vi "TestAsyncGrip.vi"() -> ()   [LabVIEW 2017]
uses:
  Projekt-RubikLibrary/ServoEnumControl.ctl
  Projekt-RubikLibrary/RubikLibraryRT.lvlib
  Projekt-RubikLibrary/RubikLibrary.lvlib
panel:
  in  "Servo 3":T1
  in  "NoWait 3":bool=TRUE
  in  "stop":bool
  in  "NoWait 2":bool=TRUE
  in  "NoWait 1":bool=TRUE
  in  "Grip closed (in)":bool
  in  "Servo 2":T1
  in  "Servo 1":T1
  # "Test Asynchronous Behaviour of Grip Servos\n\n\"Asynchronous\" means that VI(software) does not\nwait (default 500ms). Actually you will observe\nsynchronous behaviour: all three grips will move\nsynchronously. But the VI does not wait for completion \nof grip.\n\n\"NoWait==T\" means grips execute in parallel\n\"NoWait==F\" shows one grip after the other."
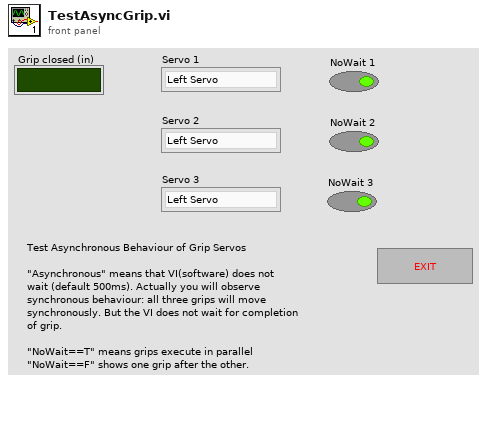
[diagram p1: front panel]
types:
  T1 = typedef "RubikLibrary.lvlib/ServoEnumControl.ctl" = enum16{"Left Servo", "Front Servo", "Right Servo"}
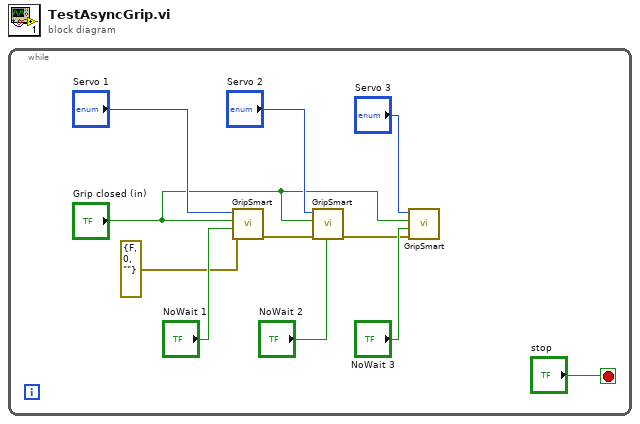
[diagram p0: block diagram]
diagram:
  n1 = while {
    stop <- "stop" stop-if-true
    n2 = call "GripSmart.vi"("error in"=errorcluster {"status"=FALSE, "code"=0, "source"=""}, "NoWait"="NoWait 1", "Grip closed (in)"="Grip closed (in)", "Servo"="Servo 1") -> ("error out"=w11:errorcluster)  [unwired: 6 in, 1 out]
    n3 = call "GripSmart.vi"("error in"=w11, "NoWait"="NoWait 2", "Grip closed (in)"="Grip closed (in)", "Servo"="Servo 2") -> ("error out"=w3:errorcluster)  [unwired: 6 in, 1 out]
    n4 = call "GripSmart.vi"("error in"=w3, "NoWait"="NoWait 3", "Grip closed (in)"="Grip closed (in)", "Servo"="Servo 3") -> ()  [unwired: 6 in, 2 out]
  }
